vi "Execute Write Request.vi"(8 "error in (no error)":errorcluster, 10 "Write Request":refnum<class "WriteRequest.lvclass">, 11 "PersistantConnectionHandler in":refnum<class "PersistantConnectionHandler.lvclass">) -> (0 "error out":errorcluster, 3 "PersistantConnectionHandler out":refnum<class "PersistantConnectionHandler.lvclass">)   [LabVIEW 2019, in "PersitantConnectionHandler.lvlib" / "PersistantConnectionHandler.lvclass"]
uses:
  <vilib>/gpm_packages/@cs/Network-interface/Source/PersistantConnectionHandler/PersistantConnectionHandler/PersistantConnectionHandler.lvclass
  C:/Program Files/National Instruments/LabVIEW 2019/vi.lib/gpm_packages/@cs/Network-interface/Source/Logged Actor/LoggedActor.lvclass
  <vilib>/gpm_packages/@cs/Network-interface/Source/MessagingInterfaces/WriteRequest/WriteRequest.lvclass
  <vilib>/gpm_packages/@cs/Network-interface/Source/PersistantConnectionHandler/PersistantConnectionHandler/PersistantConnectionHandler.lvclass/PersistantConnectionHandler.ctl
  <vilib>/gpm_packages/@cs/event-logger/Source/Composed Log/Types/Log Level.ctl
  <vilib>/gpm_packages/@cs/Network-interface/Source/Logged Actor/LoggedActor.lvclass/LoggedActor.ctl
  <vilib>/gpm_packages/@cs/event-logger/Source/Composed Log/LoggerReference/LoggerReference.lvclass/LoggerReference.ctl
  <vilib>/gpm_packages/@cs/event-logger/Source/Composed Log/LoggerReference/Log Event.vi
  <vilib>/gpm_packages/@cs/event-logger/Source/Composed Log/LoggerReference/Log.vi
  <vilib>/gpm_packages/@cs/event-logger/Source/Composed Log/LoggerReference/Get Valid Event Time.vi
  <vilib>/gpm_packages/@cs/event-logger/Source/Composed Log/LoggerReference/Remove Stale Logs.vi
  <vilib>/ErrorRing/Error Ring.xnode
  <vilib>/gpm_packages/@cs/event-logger/Source/Composed Log/Composed Log.lvlib
  <vilib>/gpm_packages/@cs/Network-interface/Source/Logged Actor/LoggedActor.lvclass
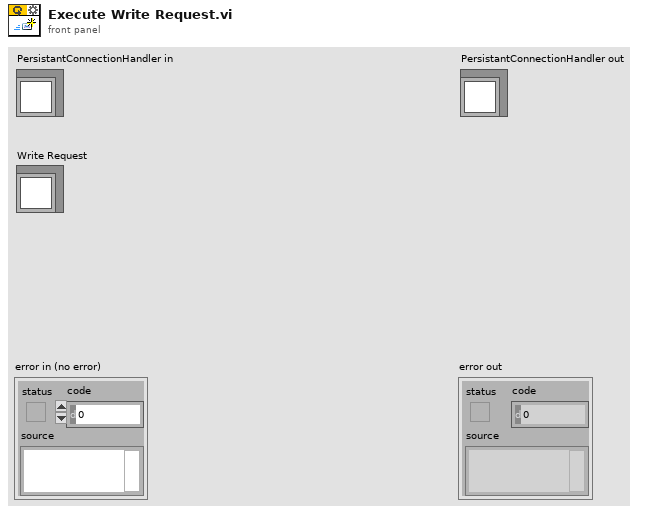
[diagram p1: front panel]
types:
  T1 = typedef "Composed Log.lvlib/Log Level.ctl" = enum16{"Debug", "Info", "Warning", "Error", "Critical"}
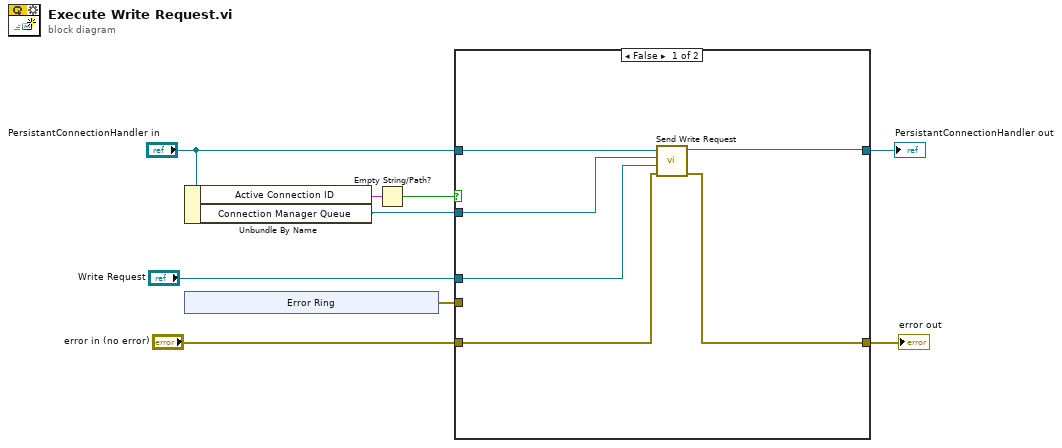
[diagram p0: block diagram]
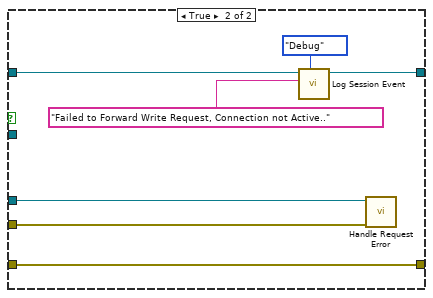
[diagram p2: hidden frame]
diagram:
  n1 = Unbundle By Name("PersistantConnectionHandler in") -> ("Active Connection ID"=w3:string, "Connection Manager Queue"=w7:refnum<class "Message Enqueuer.lvclass">)
  n2 = xnode "Error Ring"() -> ("error out"=w1:errorcluster)
  n3 = Empty String/Path?(string/path=w3) -> (empty?=w2:bool)
  n4 = case shown="False" w2 {
    tunnel: "PersistantConnectionHandler in" -> [w15 w17]
    tunnel: [w14 w16] -> w8
    tunnel: w7 -> [w13 _]
    tunnel: "error in (no error)" -> [w11 w22]
    tunnel: "Write Request" -> [w12 w21]
    tunnel: [w10 w22] -> w4
    tunnel: w1 -> [_ w20]
    frame False {
      n5 = call <vilib>:"Send Write Request.vi"("error in (no error)"=w11, "Write Request"=w12, "Connection Manager Queue"=w13, "PersistantConnectionHandler in"=w15) -> ("error out"=w10:errorcluster, "PersistantConnectionHandler out"=w14:refnum<class "PersistantConnectionHandler.lvclass">)  [unwired: 6 in]
    }
    frame True {
      n6 = call <vilib>:"Log Session Event.vi"("Event Level"=Log_Level."Debug", "Event Data"="Failed to Forward Write Request, Connection not Active..", "SessionActor in"=w17) -> ("SessionActor out"=w16:refnum<class "PersistantConnectionHandler.lvclass">)  [unwired: 7 in, 1 out]
      n7 = call-dynamic "Handle Request Error.vi"("Request Error"=w20, "WriteRequest in"=w21) -> ()  [unwired: 10 in]
    }
  }
  "error out" <- w4
  "PersistantConnectionHandler out" <- w8
